vi "AutoOff.vi"(3 "EN":bool, 4 "Old In":i32=100, 5 "Dealy (ms)":i32=100) -> (0 "Old Out":i32, 2 "Flash":bool)   [LabVIEW 2017]
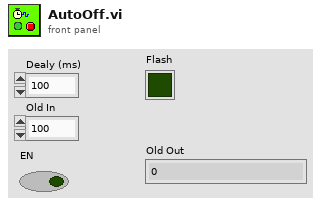
[diagram p1: front panel]
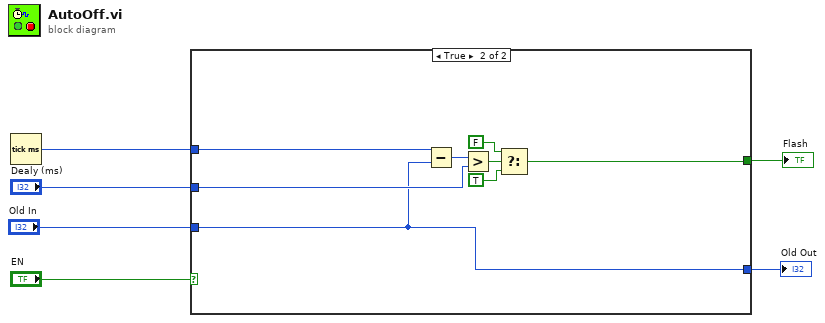
[diagram p0: block diagram]
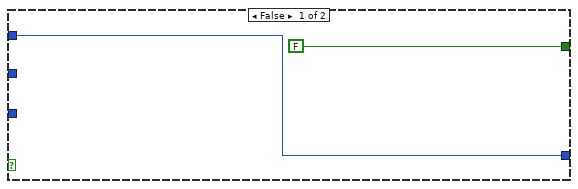
[diagram p2: hidden frame]
diagram:
  n1 = Tick Count (ms)() -> (millisecond timer value=w4:u32)
  n2 = case shown="True" "EN" {
    tunnel: "Dealy (ms)" -> [_ w16]
    tunnel: w4 -> [w7 w15]
    tunnel: [FALSE ("f") w11] -> w3
    tunnel: [w7 w9] -> w2
    tunnel: "Old In" -> [_ w9]
    frame False {
    }
    frame True {
      n3 = Subtract(x=w15, y=w9) -> (x-y=w14:u32)
      n4 = Greater?(x=w14, y=w16) -> (0:w13:bool)
      n5 = Select(t=FALSE ("Flash"), s=w13, f=TRUE) -> (s? t:f=w11:bool)
    }
  }
  "Flash" <- w3
  "Old Out" <- w2
